vi "Consolidate Whitespace Lines in Reported Error Message.vi"(1 "Reported Error In":T1) -> (0 "Reported Error Out (error message consolidated whitelines)":T1)   [LabVIEW 2016, in "Error Manager.lvlib"]
doc: "This VI consolidates (reduces) any consecutive whitespace lines in the Error message to a single whitespace line. In other words, if the error message contains two or more consecutive whitespace lines, these will be replaced with a single whitespace line.\n\n<B>Example</B>\nInput Error Message\n\"\nError Manager.lvlib:Simple Tester.lvclass:Simple Tester.vi<ERR>\ntincidunt vel nibh id tristique. Pellentesque aliquet libero rutrum tortor vulputate, quis euismod turpis blandit. Phasellus efficitur feugiat convallis. Aliquam lectus ipsum, sodales et velit vel, iaculis mollis est.\n\nUt commodo tempus elit, ac tincidunt dui vehicula et. Suspendisse convallis ante sit amet felis semper ultrices.\n\n\n<b>Complete call chain:</b>\n Error Manager.lvlib:Simple Tester.lvclass:Simple Tester.vi\n\". Notice the double whitespace line just before <b>Complete call chain:</b>\n\nOutput\n\"\nError Manager.lvlib:Simple Tester.lvclass:Simple Tester.vi<ERR>\ntincidunt vel nibh id tristique. Pellentesque aliquet libero rutrum tortor vulputate, quis euismod turpis blandit. Phasellus efficitur feugiat convallis. Aliquam lectus ipsum, sodales et velit vel, iaculis mollis est.\n\nUt commodo tempus elit, ac tincidunt dui vehicula et. Suspendisse convallis ante sit amet felis semper ultrices.\n\n<b>Complete call chain:</b>\nError Manager.lvlib:Simple Tester.lvclass:Simple Tester.vi\n\". Notice that the double whitespace line was reduced to one whitespace line."
uses:
  Error Manager.lvlib
  Public API VIs/Show Error Window Instruction (enum).ctl
  Reported Error (cluster).ctl
panel:
  # "Development\nControls or indicators that are useful for development or testing, but which are not outputs of the VI."
  # "Input\nInputs to the VI"
  # "Output\nOutputs of the VI"
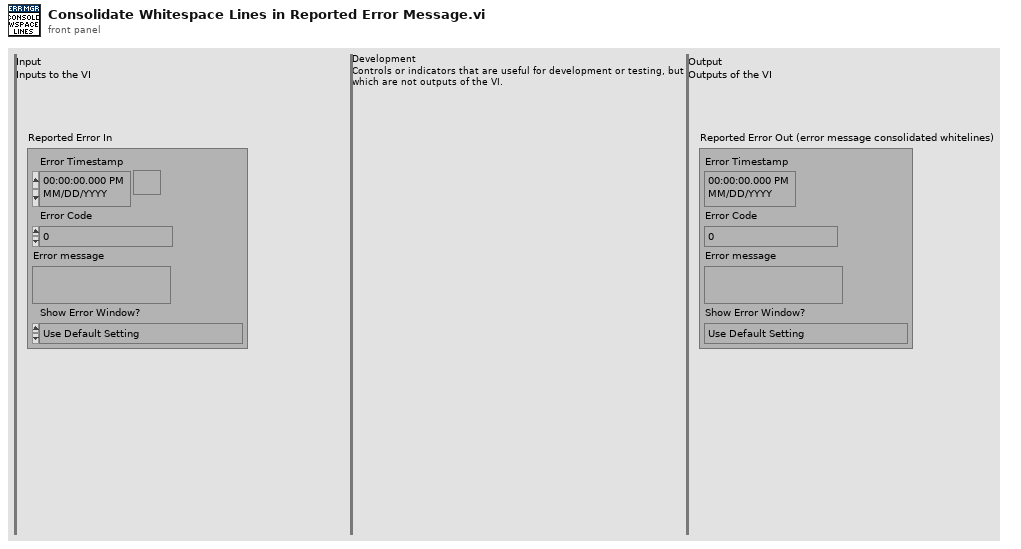
[diagram p1: front panel]
types:
  T1 = typedef "Error Manager.lvlib/Reported Error (cluster).ctl" = cluster{"Error Timestamp":timestamp, "Error Code":i32, "Error message":string, "Show Error Window?":T2}
  T2 = typedef "Error Manager.lvlib/Show Error Window Instruction (enum).ctl" = enum16{"Use Default Setting", "Show", "Do Not Show"}
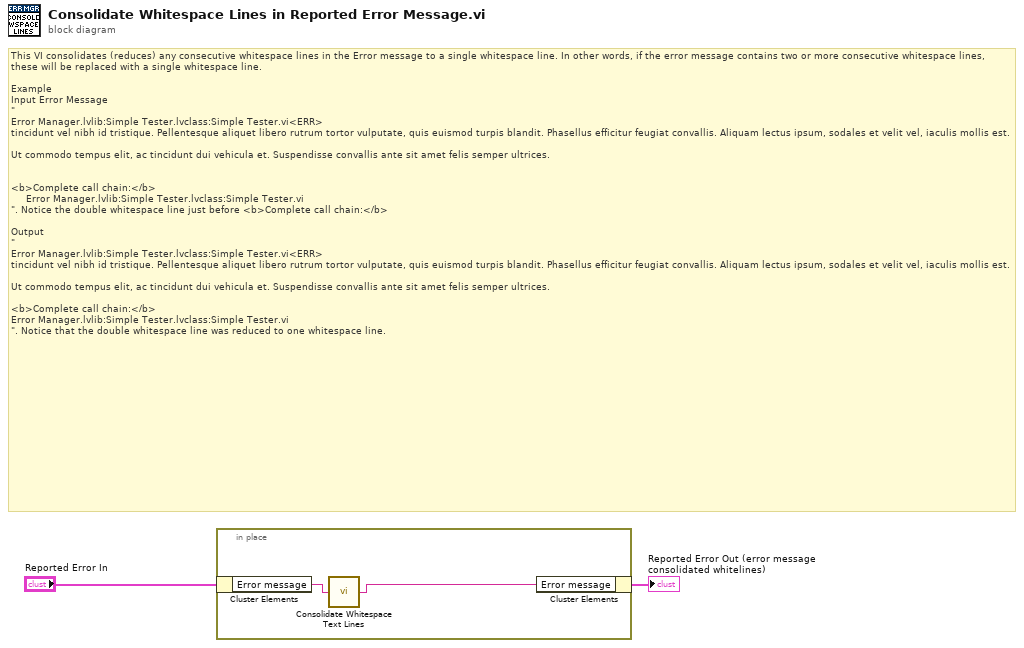
[diagram p0: block diagram]
diagram:
  # "This VI consolidates (reduces) any consecutive whitespace lines in the Error message to a single whitespace line. In other words, if the error message contains two or more consecutive whitespace lines, these will be replaced with a single whitespace line.\n\nExample\nInput Error Message\n\"\nError Manager.lvlib:Simple Tester.lvclass:Simple Tester.vi<ERR>\ntincidunt vel nibh id tristique. Pellentesque aliquet libero rutrum tortor vulputate, quis euismod turpis blandit. Phasellus efficitur feugiat convallis. Aliquam lectus ipsum, sodales et velit vel, iaculis mollis est.\n\nUt commodo tempus elit, ac tincidunt dui vehicula et. Suspendisse convallis ante sit amet felis semper ultrices.\n\n\n<b>Complete call chain:</b>\n     Error Manager.lvlib:Simple Tester.lvclass:Simple Tester.vi\n\". Notice the double whitespace line just before <b>Complete call chain:</b>\n\nOutput\n\"\nError Manager.lvlib:Simple Tester.lvclass:Simple Tester.vi<ERR>\ntincidunt vel nibh id tristique. Pellentesque aliquet libero rutrum tortor vulputate, quis euismod turpis blandit. Phasellus efficitur feugiat convallis. Aliquam lectus ipsum, sodales et velit vel, iaculis mollis est.\n\nUt commodo tempus elit, ac tincidunt dui vehicula et. Suspendisse convallis ante sit amet felis semper ultrices.\n\n<b>Complete call chain:</b>\nError Manager.lvlib:Simple Tester.lvclass:Simple Tester.vi\n\". Notice that the double whitespace line was reduced to one whitespace line."
  n1 = in-place {
    n2 = in-place-cluster #1("Reported Error In") -> ("Error message"=w4:string)
    n3 = call "Consolidate Whitespace Text Lines.vi"("Input"=w4) -> ("Output (consolidated whitespace lines)"=w3:string)
    n4 = in-place-cluster #1("Error message"=w3) -> (→"Reported Error Out (error message consolidated whitelines)":T1)
  }
